vi "myRIO__TCP_constants_byteRange_messageType_selectResponse.vi"() -> (2 "output_selResponse_byte":u8=82, 3 "output_selectResponse_char":string="R")   [LabVIEW 2014]
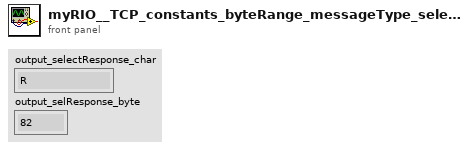
[diagram p1: front panel]
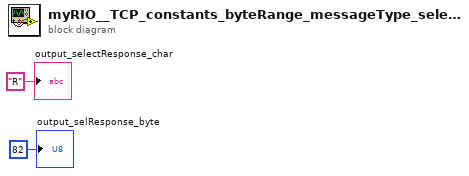
[diagram p0: block diagram]
diagram:
  "output_selectResponse_char" <- "R"
  "output_selResponse_byte" <- u8 82
